vi "Config OK Tab.vi"(8 "error in (no error)":errorcluster, 9 "String Selected":T1, 11 "Rigol DG822 Sine in":refnum<class "Rigol DG822 Sine.lvclass">) -> (0 "error out":errorcluster, 3 "Rigol DG822 Sine out":refnum<class "Rigol DG822 Sine.lvclass">)   [LabVIEW 2021, in "Rigol DG822 UI.lvlib" / "Rigol DG822 Sine.lvlib" / "Rigol DG822 Sine.lvclass"]
uses:
  Rigol DG822 Sine.lvclass
  Rigol DG822 UI/lib/controls.llb/StringIndicatorSelected.ctl
  Rigol DG822 Sine.lvclass/Rigol DG822 Sine.ctl
  General/Files/lvlibp/Actors.lvlibp/Actors/Actors/Actors.lvclass
  D:/LabVIEW/General/Files/lvlibp/Actors.lvlibp/Actors/Actors/Actors.lvclass
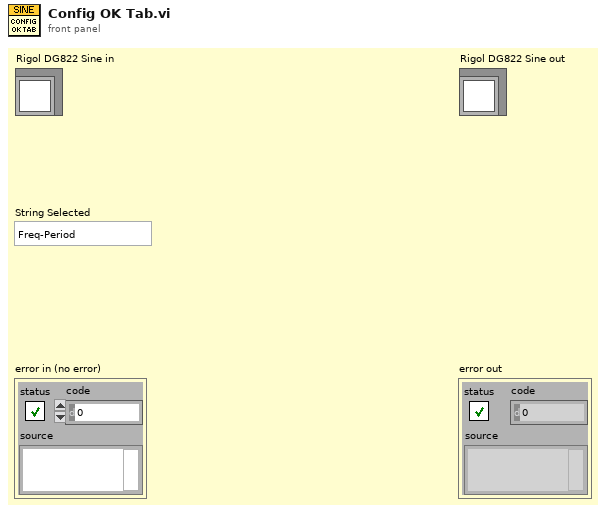
[diagram p1: front panel]
types:
  T1 = typedef "StringIndicatorSelected.ctl" = enum16{"Freq-Period", "Ampl-HighL", "Offset-LowL", "Phase", "Duty-Width", "RisEdge", "FallEdge"}
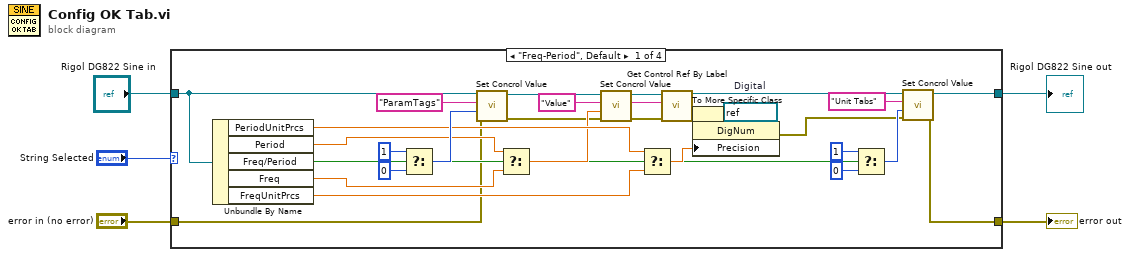
[diagram p0: block diagram]
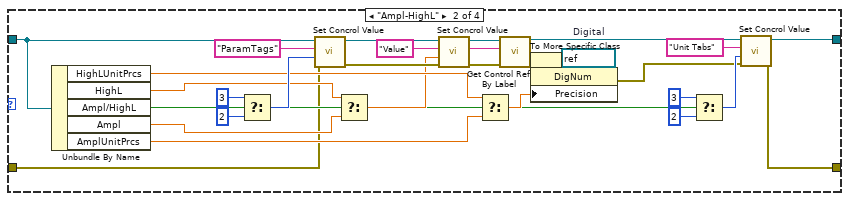
[diagram p2: hidden frame]
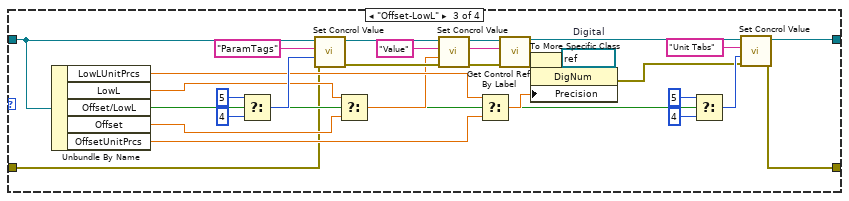
[diagram p3: hidden frame]
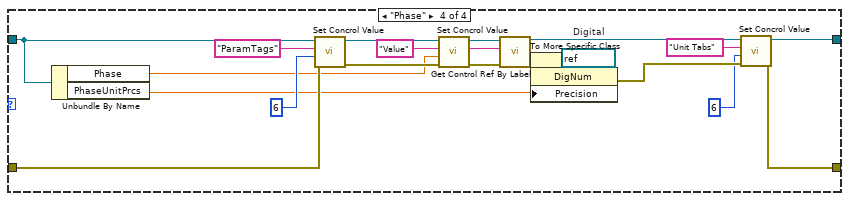
[diagram p4: hidden frame]
diagram:
  n1 = case shown="\"Freq-Period\", Default" "String Selected" {
    tunnel: [w12 w41 w72 w106] -> w5
    tunnel: "Rigol DG822 Sine in" -> [w7 w54 w85 w113]
    tunnel: [w8 w37 w68 w103] -> w2
    tunnel: "error in (no error)" -> [w9 w38 w69 w104]
    frame "Freq-Period", Default {
      w29 = refnum<vi> refnum  # Digital
      w20 = "Value" ("Control Label")
      n2 = Unbundle By Name(w7) -> ("PeriodUnitPrcs"=w15:dbl, "Period"=w18:dbl, "Freq/Period"=w10:bool, "Freq"=w17:dbl, "FreqUnitPrcs"=w16:dbl)
      n3 = Select(t=u16 1 ("ParamTags"), s=w10, f=u16 0 ("ParamTags")) -> (s? t:f=w21:u16)
      n4 = call "Set Concrol Value.vi"("error in (no error)"=w9, "Value"=w21, "Control Label"="ParamTags", "Actors in"=w7) -> ("error out"=w6:errorcluster, "Actors out"=w23:refnum<class "Rigol DG822 Sine.lvclass">)  [unwired: 6 in]
      n5 = Select(t=w18, s=w10, f=w17) -> (s? t:f=w14:dbl)
      n6 = call "Set Concrol Value.vi"("error in (no error)"=w6, "Value"=w14, "Control Label"=w20, "Actors in"=w23) -> ("error out"=w19:errorcluster, "Actors out"=w22:refnum<class "Rigol DG822 Sine.lvclass">)  [unwired: 6 in]
      n7 = Select(t=w15, s=w10, f=w16) -> (s? t:f=w30:dbl)
      n8 = call "Get Control Ref By Label.vi"("error in (no error)"=w19, "Control Label"=w20, "Actors in"=w22) -> ("error out"=w31:errorcluster, "Control Ref"=w27:refnum<vi>, "Actors out"=w13:refnum<class "Rigol DG822 Sine.lvclass">)  [unwired: 6 in]
      n9 = To More Specific Class(target class=w29, reference=w27, error in=w31) -> (specific class reference=w28:refnum<vi>, error out=w32:errorcluster)
      n10 = property class="DigNum"(reference=w28, error in=w32, "Precision"=w30) -> (error out=w11:errorcluster)  [unwired: 1 out]
      n11 = Select(t=u16 1 ("ParamTags"), s=w10, f=u16 0 ("ParamTags")) -> (s? t:f=w36:u16)
      n12 = call "Set Concrol Value.vi"("error in (no error)"=w11, "Value"=w36, "Control Label"="Unit Tabs", "Actors in"=w13) -> ("error out"=w8:errorcluster, "Actors out"=w12:refnum<class "Rigol DG822 Sine.lvclass">)  [unwired: 6 in]
    }
    frame "Ampl-HighL" {
      w60 = refnum<vi> refnum  # Digital
      w50 = "Value" ("Control Label")
      n13 = Unbundle By Name(w54) -> ("HighLUnitPrcs"=w44:dbl, "HighL"=w47:dbl, "Ampl/HighL"=w39:bool, "Ampl"=w46:dbl, "AmplUnitPrcs"=w45:dbl)
      n14 = Select(t=u16 3 ("ParamTags"), s=w39, f=u16 2 ("ParamTags")) -> (s? t:f=w51:u16)
      n15 = call "Set Concrol Value.vi"("error in (no error)"=w38, "Value"=w51, "Control Label"="ParamTags", "Actors in"=w54) -> ("error out"=w49:errorcluster, "Actors out"=w53:refnum<class "Rigol DG822 Sine.lvclass">)  [unwired: 6 in]
      n16 = Select(t=w47, s=w39, f=w46) -> (s? t:f=w43:dbl)
      n17 = call "Set Concrol Value.vi"("error in (no error)"=w49, "Value"=w43, "Control Label"=w50, "Actors in"=w53) -> ("error out"=w48:errorcluster, "Actors out"=w52:refnum<class "Rigol DG822 Sine.lvclass">)  [unwired: 6 in]
      n18 = Select(t=w44, s=w39, f=w45) -> (s? t:f=w61:dbl)
      n19 = call "Get Control Ref By Label.vi"("error in (no error)"=w48, "Control Label"=w50, "Actors in"=w52) -> ("error out"=w62:errorcluster, "Control Ref"=w58:refnum<vi>, "Actors out"=w42:refnum<class "Rigol DG822 Sine.lvclass">)  [unwired: 6 in]
      n20 = To More Specific Class(target class=w60, reference=w58, error in=w62) -> (specific class reference=w59:refnum<vi>, error out=w63:errorcluster)
      n21 = property class="DigNum"(reference=w59, error in=w63, "Precision"=w61) -> (error out=w40:errorcluster)  [unwired: 1 out]
      n22 = Select(t=u16 3 ("ParamTags"), s=w39, f=u16 2 ("ParamTags")) -> (s? t:f=w67:u16)
      n23 = call "Set Concrol Value.vi"("error in (no error)"=w40, "Value"=w67, "Control Label"="Unit Tabs", "Actors in"=w42) -> ("error out"=w37:errorcluster, "Actors out"=w41:refnum<class "Rigol DG822 Sine.lvclass">)  [unwired: 6 in]
    }
    frame "Offset-LowL" {
      w91 = refnum<vi> refnum  # Digital
      w81 = "Value" ("Control Label")
      n24 = Unbundle By Name(w85) -> ("LowLUnitPrcs"=w75:dbl, "LowL"=w78:dbl, "Offset/LowL"=w70:bool, "Offset"=w77:dbl, "OffsetUnitPrcs"=w76:dbl)
      n25 = Select(t=u16 5 ("ParamTags"), s=w70, f=u16 4 ("ParamTags")) -> (s? t:f=w82:u16)
      n26 = call "Set Concrol Value.vi"("error in (no error)"=w69, "Value"=w82, "Control Label"="ParamTags", "Actors in"=w85) -> ("error out"=w80:errorcluster, "Actors out"=w84:refnum<class "Rigol DG822 Sine.lvclass">)  [unwired: 6 in]
      n27 = Select(t=w78, s=w70, f=w77) -> (s? t:f=w74:dbl)
      n28 = call "Set Concrol Value.vi"("error in (no error)"=w80, "Value"=w74, "Control Label"=w81, "Actors in"=w84) -> ("error out"=w79:errorcluster, "Actors out"=w83:refnum<class "Rigol DG822 Sine.lvclass">)  [unwired: 6 in]
      n29 = Select(t=w75, s=w70, f=w76) -> (s? t:f=w92:dbl)
      n30 = call "Get Control Ref By Label.vi"("error in (no error)"=w79, "Control Label"=w81, "Actors in"=w83) -> ("error out"=w93:errorcluster, "Control Ref"=w89:refnum<vi>, "Actors out"=w73:refnum<class "Rigol DG822 Sine.lvclass">)  [unwired: 6 in]
      n31 = To More Specific Class(target class=w91, reference=w89, error in=w93) -> (specific class reference=w90:refnum<vi>, error out=w94:errorcluster)
      n32 = property class="DigNum"(reference=w90, error in=w94, "Precision"=w92) -> (error out=w71:errorcluster)  [unwired: 1 out]
      n33 = Select(t=u16 5 ("ParamTags"), s=w70, f=u16 4 ("ParamTags")) -> (s? t:f=w98:u16)
      n34 = call "Set Concrol Value.vi"("error in (no error)"=w71, "Value"=w98, "Control Label"="Unit Tabs", "Actors in"=w73) -> ("error out"=w68:errorcluster, "Actors out"=w72:refnum<class "Rigol DG822 Sine.lvclass">)  [unwired: 6 in]
    }
    frame "Phase" {
      w117 = refnum<vi> refnum  # Digital
      w110 = "Value" ("Control Label")
      n35 = Unbundle By Name(w113) -> ("Phase"=w101:dbl, "PhaseUnitPrcs"=w100:dbl)
      n36 = call "Set Concrol Value.vi"("error in (no error)"=w104, "Value"=u16 6 ("ParamTags"), "Control Label"="ParamTags", "Actors in"=w113) -> ("error out"=w109:errorcluster, "Actors out"=w112:refnum<class "Rigol DG822 Sine.lvclass">)  [unwired: 6 in]
      n37 = call "Set Concrol Value.vi"("error in (no error)"=w109, "Value"=w101, "Control Label"=w110, "Actors in"=w112) -> ("error out"=w108:errorcluster, "Actors out"=w111:refnum<class "Rigol DG822 Sine.lvclass">)  [unwired: 6 in]
      n38 = call "Get Control Ref By Label.vi"("error in (no error)"=w108, "Control Label"=w110, "Actors in"=w111) -> ("error out"=w118:errorcluster, "Control Ref"=w115:refnum<vi>, "Actors out"=w107:refnum<class "Rigol DG822 Sine.lvclass">)  [unwired: 6 in]
      n39 = To More Specific Class(target class=w117, reference=w115, error in=w118) -> (specific class reference=w116:refnum<vi>, error out=w119:errorcluster)
      n40 = property class="DigNum"(reference=w116, error in=w119, "Precision"=w100) -> (error out=w105:errorcluster)  [unwired: 1 out]
      n41 = call "Set Concrol Value.vi"("error in (no error)"=w105, "Value"=u16 6 ("ParamTags"), "Control Label"="Unit Tabs", "Actors in"=w107) -> ("error out"=w103:errorcluster, "Actors out"=w106:refnum<class "Rigol DG822 Sine.lvclass">)  [unwired: 6 in]
    }
  }
  "error out" <- w2
  "Rigol DG822 Sine out" <- w5
